vi "外部交互全局.vi"() -> ()   [LabVIEW 2016, in "数据传输系统-03.lvlib"]
panel:
  in  "数据库ID秘钥":cluster{"userID":string, "password":string}
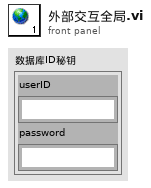
[diagram p1: front panel]
diagram:
